vi "Results.Evaluate Overall Result Based on Failure Priority.vi"(9 "ConfigDir":path, 11 "Meas":T3[](array[typedef]) {"Status" items=["LOG", "PASS", "FAIL", "ERROR"]}) -> (2 "Change":bool, 3 "ResultState":T1={"State"=enum."Passing", "Code"=0, "Description"=""})   [LabVIEW 2018]
uses:
  Result.Measurement Item.ctl
  Result.Measurement and Attribute Item Status.ctl
  <vilib>/KATE/SeqMgr/SeqMgr.Result Info.ctl
  <vilib>/KATE/SeqMgr/SeqMgr.Result State Enum.ctl
  <vilib>/KATE/SeqMgr/SeqMgr.lvlib
  <vilib>/KATE/Files/File Utils.lvlib
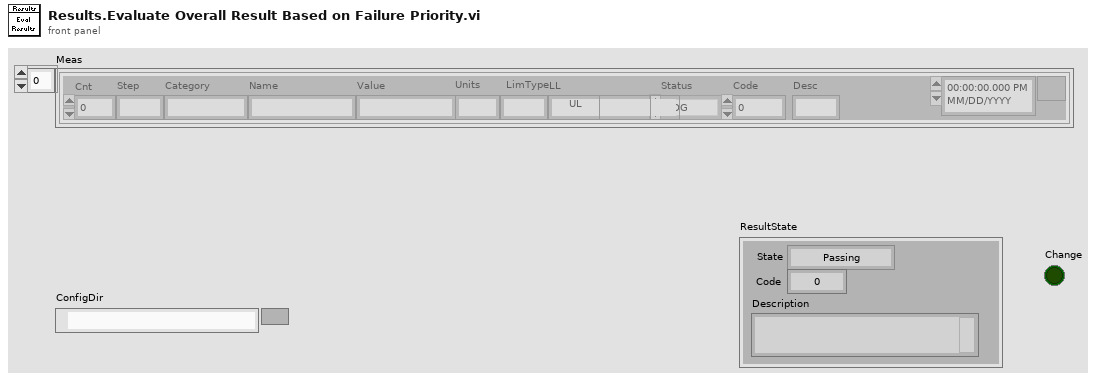
[diagram p1: front panel]
types:
  T1 = typedef "KATE_Lib.lvlib/SeqMgr.lvlib/SeqMgr.Result Info.ctl" = cluster{"State":T2, "Code":i32, "Description":string}
  T2 = typedef "KATE_Lib.lvlib/SeqMgr.lvlib/SeqMgr.Result State Enum.ctl" = enum16{"None", "Passing", "Failing", "PASS", "FAIL", "ABORT", "ERROR"}
  T3 = typedef "Result.Measurement Item.ctl" = cluster{"Cnt":i32, "Step":string, "Category":string, "Name":string, "Value":string, "Units":string, "LimType":string, "LL":string, "UL":string, "Status":T4, "Code":i32, "Desc":string, "Time":timestamp}
  T4 = typedef "Result.Measurement and Attribute Item Status.ctl" = i32
  T5 = cluster{"Names":string[], "Status":T4[], "Codes":i32[], "Descs":string[]}
  T6 = cluster{"Results":cluster{"Names":string[], "Status":T4[], "Codes":i32[], "Descs":string[]}, "Pri":cluster{"Names":string[], "Status":T2[]}}
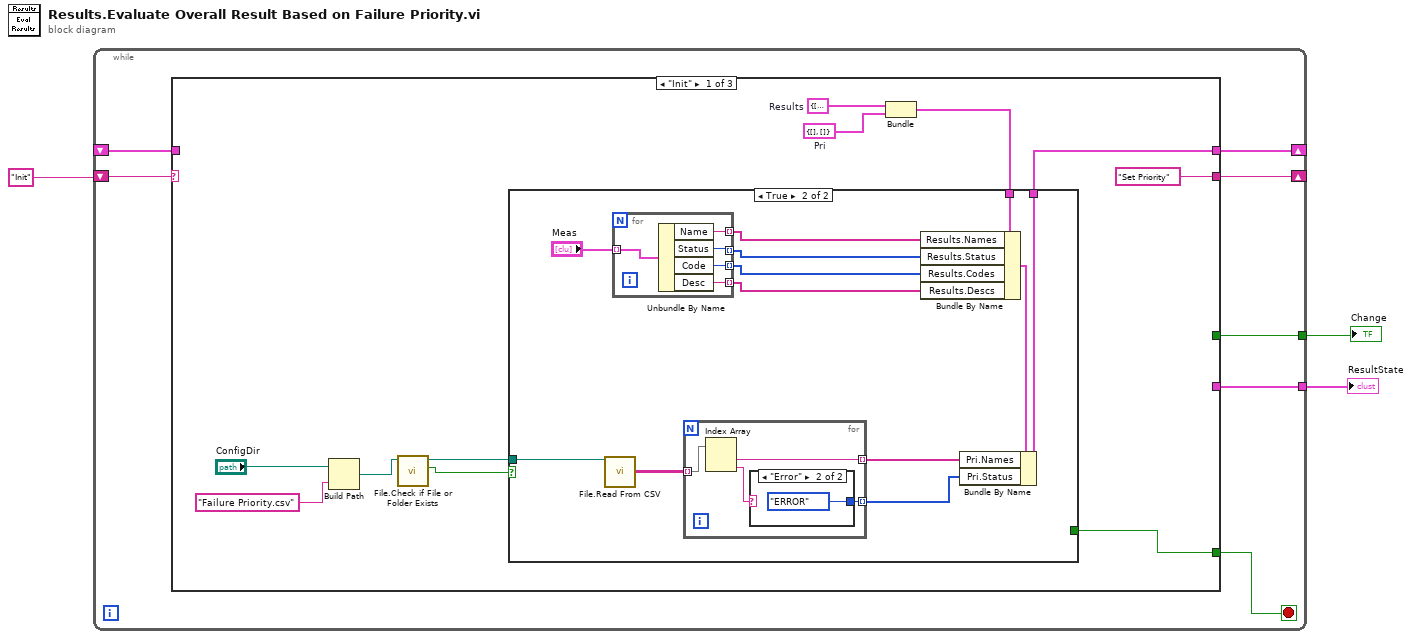
[diagram p0: block diagram]
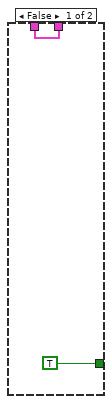
[diagram p2: hidden frame]
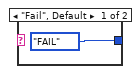
[diagram p3: hidden frame]
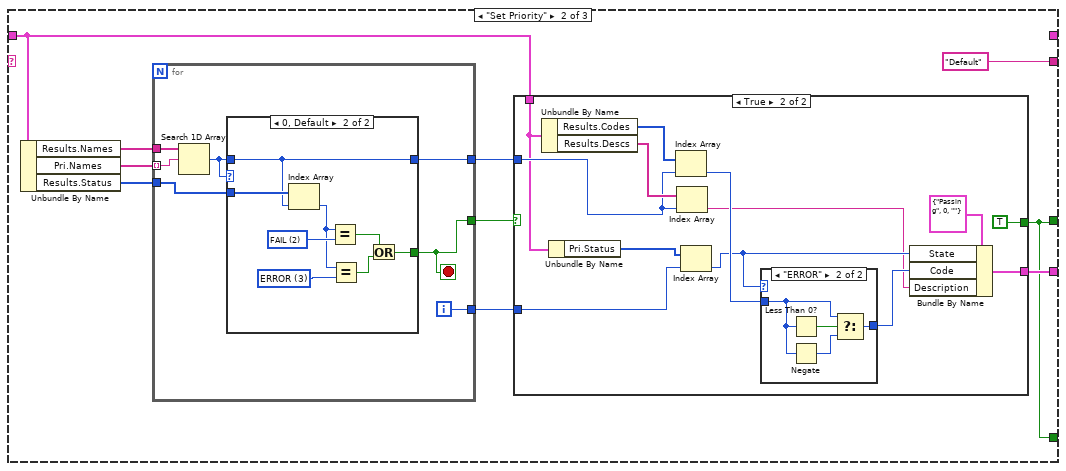
[diagram p4: hidden frame]
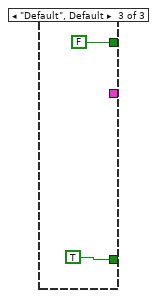
[diagram p8: hidden frame]
diagram:
  n1 = while {
    shift-right: [w9] -> _
    shift-left: "Init" -> [w10]
    tunnel: [w7] -> w2
    tunnel: [w6] -> w1
    shift-right: [w4] -> _
    shift-left: _ -> [w5]
    stop <- w8 stop-if-true
    n2 = case shown="\"Init\"" w10 {
      tunnel: ["Set Priority" "Default" _] -> w9
      tunnel: [w11 w54 TRUE] -> w8
      tunnel: [_ w54 FALSE] -> w7
      tunnel: [_ w55 _] -> w6
      tunnel: w5 -> [_ w49 _]
      tunnel: [w15 _ _] -> w4
      frame "Init" {
        w17 = cluster{"Names":string[], "Status":T2[]} {"Names"=[], "Status"=[]}  # Pri
        w18 = T5 {"Names"=[], "Status"=[], "Codes"=[], "Descs"=[]}  # Results
        n3 = Build Path(base path="ConfigDir", name or relative path="Failure Priority.csv") -> (appended path=w14:path)
        n4 = call <vilib>:"File.Check if File or Folder Exists.vi"("Path"=w14) -> ("Exists"=w12:bool, "Dup Path"=w13:path)  [unwired: 6 in, 3 out]
        n5 = Bundle("Results"=w18, "Pri"=w17) -> (w16:T6)  [unwired: 1 in]
        n6 = case shown="True" w12 {
          tunnel: w16 -> [w23 w31]
          tunnel: [w23 w29] -> w15
          tunnel: w13 -> [_ w24]
          tunnel: [TRUE _] -> w11
          frame False {
          }
          frame True {
            n7 = call <vilib>:"File.Read From CSV.vi"("File"=w24) -> ("Data"=w28:string[][])  [unwired: 8 in, 2 out]
            n8 = for {
              tunnel: "Meas" -> [w46] mode=indexing
              tunnel: [w45] -> w35 mode=indexing
              tunnel: [w44] -> w34 mode=indexing
              tunnel: [w43] -> w33 mode=indexing
              tunnel: [w42] -> w32 mode=indexing
              n9 = Unbundle By Name(w46) -> ("Name"=w45:string, "Status"=w44:T4, "Code"=w43:i32, "Desc"=w42:string)
            }
            n10 = for {
              tunnel: w28 -> [w39] mode=indexing
              tunnel: [w38] -> w27 mode=indexing
              tunnel: [w36] -> w26 mode=indexing
              n11 = Index Array(array=w39) -> (element #1=w38:string, element #2=w37:string)  [unwired: 2 in]
              n12 = case shown="\"Error\"" w37 {
                tunnel: [SeqMgr.Result_State_Enum."FAIL" ("State") SeqMgr.Result_State_Enum."ERROR" ("State")] -> w36
                frame "Fail", Default {
                }
                frame "Error" {
                }
              }
            }
            n13 = Bundle By Name(cluster=w31, "Results.Names"=w35, "Results.Status"=w34, "Results.Codes"=w33, "Results.Descs"=w32) -> (w30:T6)
            n14 = Bundle By Name(cluster=w30, "Pri.Names"=w27, "Pri.Status"=w26) -> (w29:T6)
          }
        }
      }
      frame "Set Priority" {
        n15 = Unbundle By Name(w49) -> ("Results.Names"=w52:string[], "Pri.Names"=w51:string[], "Results.Status"=w50:T4[])
        n16 = for {
          tunnel: [w59] -> w53
          tunnel: w52 -> [w63]
          tunnel: w51 -> [w62] mode=indexing
          tunnel: w50 -> [w61]
          tunnel: [w58] -> w48
          tunnel: [w57] -> w47
          i -> [w57]
          stop <- w59 stop-if-true
          n17 = Search 1D Array(1D array=w63, element=w62) -> (index of element=w60:i32)  [unwired: 1 in]
          n18 = case shown="0, Default" w60 {
            tunnel: w60 -> [_ w64]
            tunnel: w61 -> [_ w70]
            tunnel: [_ w65] -> w59
            tunnel: [_ w64] -> w58
            frame -1 {
            }
            frame 0, Default {
              w68 = T4 3 items=["LOG", "PASS", "FAIL", "ERROR"] ("y")
              w71 = T4 2 items=["LOG", "PASS", "FAIL", "ERROR"] ("y")
              n19 = Index Array(array=w70, index=w64) -> (element=w69:T4)
              n20 = Equal?(x=w69, y=w71) -> (x = y?=w67:bool)
              n21 = Equal?(x=w69, y=w68) -> (x = y?=w66:bool)
              n22 = Or(x=w67, y=w66) -> (x .or. y?=w65:bool)
            }
          }
        }
        n23 = case shown="True" w53 {
          tunnel: [_ w83] -> w55
          tunnel: [_ TRUE] -> w54
          tunnel: w49 -> [_ w77]
          tunnel: w48 -> [_ w78]
          tunnel: w47 -> [_ w75]
          frame False {
          }
          frame True {
            n24 = Unbundle By Name(w77) -> ("Results.Codes"=w80:i32[], "Results.Descs"=w79:string[])
            n25 = Unbundle By Name(w77) -> ("Pri.Status"=w76:T2[])
            n26 = Index Array(array=w80, index=w78) -> (element=w74:i32)
            n27 = Index Array(array=w79, index=w78) -> (element=w72:string)
            n28 = Index Array(array=w76, index=w75) -> (element=w73:T2)
            n29 = case shown="\"ERROR\"" w73 {
              tunnel: [w85 w87] -> w81
              tunnel: w74 -> [w85 w86]
              frame Default {
              }
              frame "ERROR" {
                n30 = Less Than 0?(x=w86) -> (x < 0?=w89:bool)
                n31 = Negate(x=w86) -> (-x=w88:i32)
                n32 = Select(t=w86, s=w89, f=w88) -> (s? t:f=w87:i32)
              }
            }
            n33 = Bundle By Name(cluster=T1 {"State"=enum."Passing", "Code"=0, "Description"=""} ("ResultState"), "State"=w73, "Code"=w81, "Description"=w72) -> (w83:T1)
          }
        }
      }
      frame "Default", Default {
      }
    }
  }
  "ResultState" <- w1
  "Change" <- w2
